vi "Vision Driving Commands.vi"(5 "Vision Mode":T1, 6 "error in (no error)":errorcluster, 7 "Number of Matches":i32, 8 "Vision Enabled":bool, 9 "Centerpoint Target":sgl=160.0, 10 "PID gains":T2={"proportional gain (Kc)"=1.0, "integral time (Ti, min)"=0.01, "derivative time (Td, min)"=0.0} {"derivative time (Td, min)" format="%.3f"; "integral time (Ti, min)" format="%.3f"; "proportional gain (Kc)" format="%.3f"}, 11 "Shape Report (calibrated)":T3(array[cluster])) -> (2 "Width":i32, 3 "Centroid.x":sgl)   [LabVIEW 2019]
uses:
  Vision Mode.ctl
  <vilib>/Rock Robotics/Network Tables/NT Write Number.vi
  <vilib>/addons/control/pid/pid.llb/PID (DBL).vi
  <vilib>/Rock Robotics/Network Tables/NT Write Numeric Array.vi
  <vilib>/addons/control/pid/NI_PID_pid.lvlib
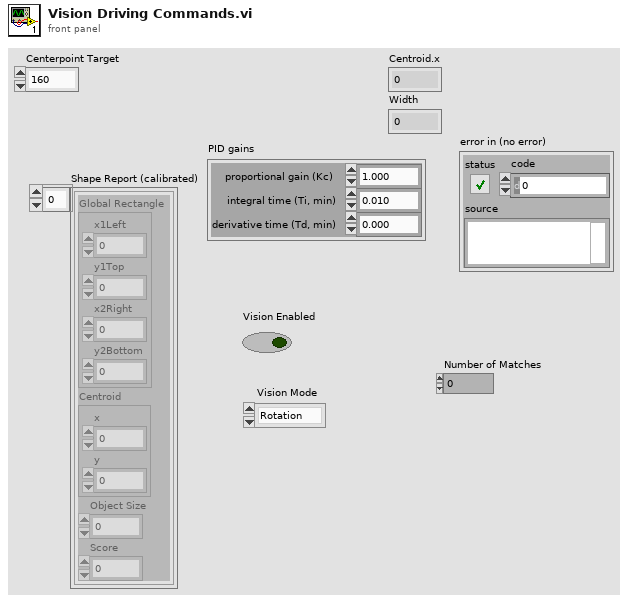
[diagram p1: front panel]
types:
  T1 = typedef "Vision Mode.ctl" = enum16{"Rotation", "Translation"}
  T2 = cluster{"proportional gain (Kc)":dbl, "integral time (Ti, min)":dbl, "derivative time (Td, min)":dbl}
  T3 = cluster{"Global Rectangle":cluster{"x1Left":i32, "y1Top":i32, "x2Right":i32, "y2Bottom":i32}, "Centroid":cluster{"x":sgl, "y":sgl}, "Object Size":u32, "Score":dbl}[]
  T4 = cluster{"Global Rectangle":cluster{"x1Left":i32, "y1Top":i32, "x2Right":i32, "y2Bottom":i32}, "Centroid":cluster{"x":sgl, "y":sgl}, "Object Size":u32, "Score":dbl}
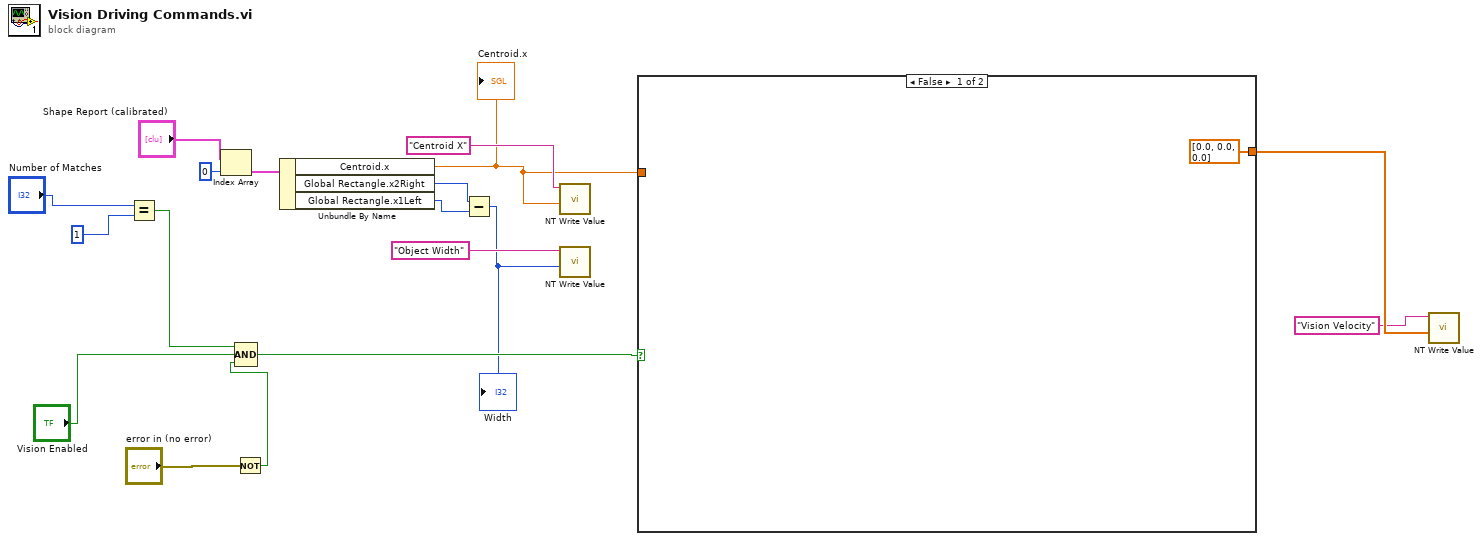
[diagram p0: block diagram]
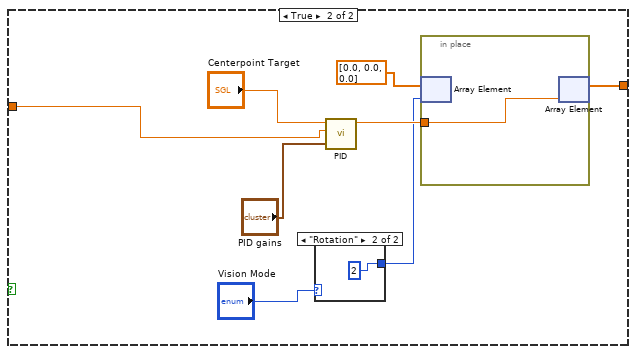
[diagram p2: hidden frame]
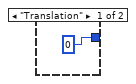
[diagram p3: hidden frame]
diagram:
  n1 = Equal?(x="Number of Matches", y=1) -> (x = y?=w9:bool)
  n2 = Index Array(array="Shape Report (calibrated)", index=0) -> (element=w15:T4)
  n3 = Not(x="error in (no error)") -> (.not. x?=w7:bool)
  n4 = Compound Arithmetic op=AND(w9, "Vision Enabled", w7) -> (w6:bool)
  n5 = Unbundle By Name(w15) -> ("Centroid.x"=w13:sgl, "Global Rectangle.x2Right"=w5:i32, "Global Rectangle.x1Left"=w4:i32)
  "Centroid.x" <- w13
  n6 = Subtract(x=w5, y=w4) -> (x-y=w3:i32)
  "Width" <- w3
  n7 = call-poly <vilib>:"NT Write Value.vi"("Numeric"=w13, "Name"="Centroid X") -> ()  [unwired: 9 in, 1 out]
  n8 = call-poly <vilib>:"NT Write Value.vi"("Numeric"=w3, "Name"="Object Width") -> ()  [unwired: 9 in, 1 out]
  n9 = case shown="False" w6 {
    tunnel: w13 -> [_ w27]
    tunnel: [dbl[] [0.0, 0.0, 0.0] ("output") w20] -> w2
    frame False {
    }
    frame True {
      n10 = case shown="\"Rotation\"" "Vision Mode" {
        tunnel: [0 2] -> w21
        frame "Translation" {
        }
        frame "Rotation" {
        }
      }
      n11 = call-poly <vilib>:"PID.vi"("PID gains"="PID gains", "process variable"=w27, "setpoint"="Centerpoint Target") -> ("output"=w22:dbl)  [unwired: 7 in, 1 out]
      n12 = in-place {
        in-place-border: w22 -> [w30]
        n13 = in-place-array #1(dbl[] [0.0, 0.0, 0.0] ("output"), w21) -> ()  [unwired: 1 out]
        n14 = in-place-array #1(w30) -> (w20:dbl[])  [unwired: 1 out]
      }
    }
  }
  n15 = call-poly <vilib>:"NT Write Value.vi"("Numeric Array"=w2, "Name"="Vision Velocity") -> ()  [unwired: 9 in, 1 out]
